vi "AndorTemperatureFGV.vi"(0 "AndorTemperature 0":T1=enum."Temperature OK", 5 "AndorTemperature 1":T1=enum."Temperature OK", 7 "Set_Get":enum16{"Set", "Get"}(ring), 9 "temperatureValues":i32[](array[numeric]), 11 "error in":errorcluster) -> (4 "Andor 0 Temperature":T1=enum."Temperature OK", 6 "Andor 1 Temperature":T1=enum."Temperature OK", 8 "temperatureValuesOut":i32[](array[numeric]), 15 "error out":errorcluster)   [LabVIEW 2010]
uses:
  controls/ctlSeqFNs_Andor_temp.ctl
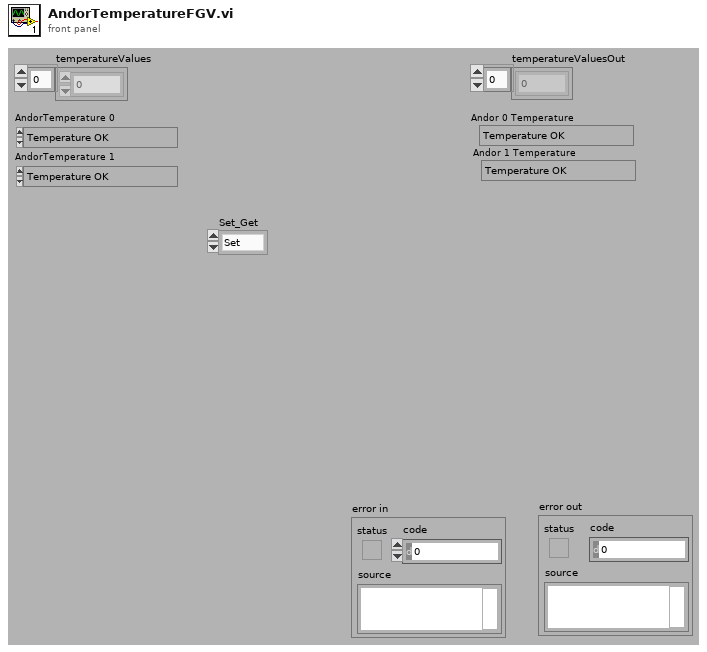
[diagram p1: front panel]
types:
  T1 = typedef "ctlSeqFNs_Andor_temp.ctl" = enum16{"Temperature  FALSE", "Temperature OK"}
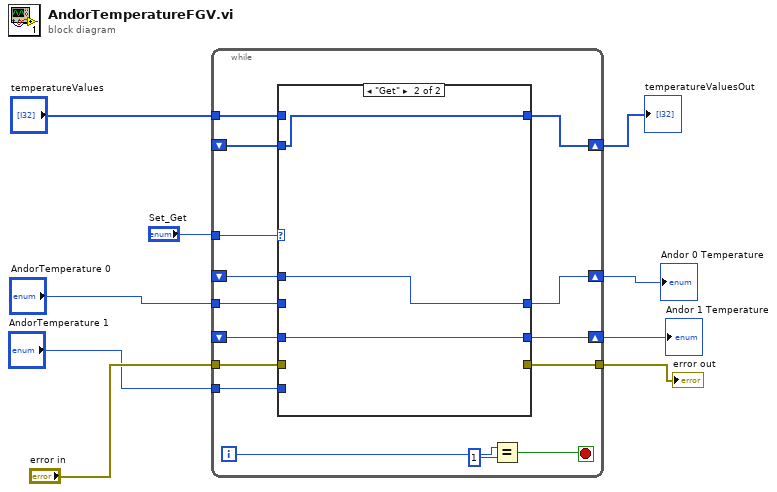
[diagram p0: block diagram]
diagram:
  n1 = while {
    tunnel: "Set_Get" -> [w24]
    tunnel: "AndorTemperature 0" -> [w23]
    shift-right: [w22] -> w7
    shift-left: _ -> [w21]
    tunnel: "error in" -> [w17]
    tunnel: [w16] -> w5
    tunnel: "AndorTemperature 1" -> [w14]
    shift-right: [w15] -> w4
    shift-left: _ -> [w13]
    shift-right: [w12] -> w2
    shift-left: _ -> [w10]
    tunnel: "temperatureValues" -> [w11]
    i -> [w19]
    stop <- w20 stop-if-true
    n2 = case shown="\"Get\"" w24 {
      tunnel: w23 -> [w28 _]
      tunnel: [w28 w31] -> w22
      tunnel: w21 -> [_ w31]
      tunnel: w17 -> [w27 _]
      tunnel: [w27 _] -> w16
      tunnel: [w26 w30] -> w15
      tunnel: w14 -> [w26 _]
      tunnel: w13 -> [_ w30]
      tunnel: w11 -> [w25 _]
      tunnel: [w25 w29] -> w12
      tunnel: w10 -> [_ w29]
      frame "Set", Default {
      }
      frame "Get" {
      }
    }
    n3 = Equal?(x=w19, y=1) -> (x = y?=w20:bool)
  }
  "Andor 0 Temperature" <- w7
  "error out" <- w5
  "Andor 1 Temperature" <- w4
  "temperatureValuesOut" <- w2
